vi "AUTON_Index.vi"(0 "Auton Array":dbl[][](array[numeric]), 5 "MeasuredHeading":dbl, 7 "LeftEncoder":dbl, 9 "RightEncoder":dbl, 11 "Kinect Array":dbl[](array[numeric])) -> (3 "Kinect Array Out":dbl[](array[numeric]), 4 "Left Drive":dbl, 6 "Right Drive":dbl)   [LabVIEW 2012]
uses:
  <vilib>/addons/Kinect/Skeleton Vertex Index.ctl
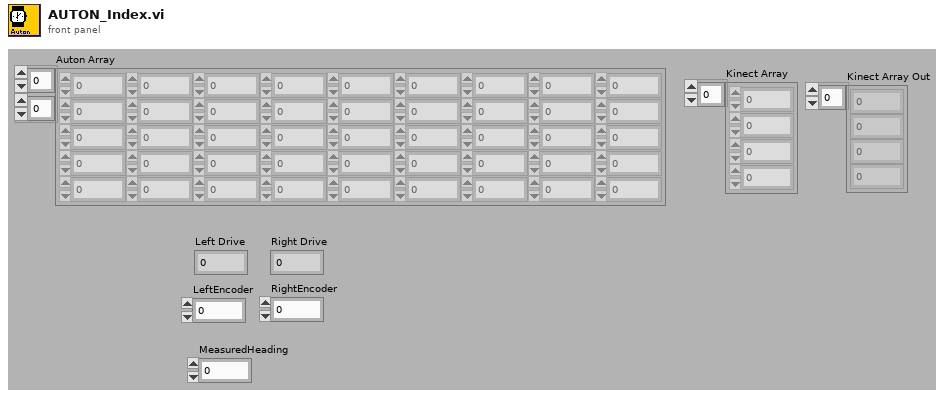
[diagram p1: front panel]
types:
  T1 = typedef "Skeleton Vertex Index.ctl" = i32
  T2 = cluster{"RightAxis":dbl, "LeftAxis":dbl, "RightHead":bool, "Left Head":bool, "Left Leg Out":bool, "Left Leg Forward":bool, "Left Leg Back":bool, "Right Leg Out":bool, "Right Leg Forward":bool, "Right Leg Back":bool}
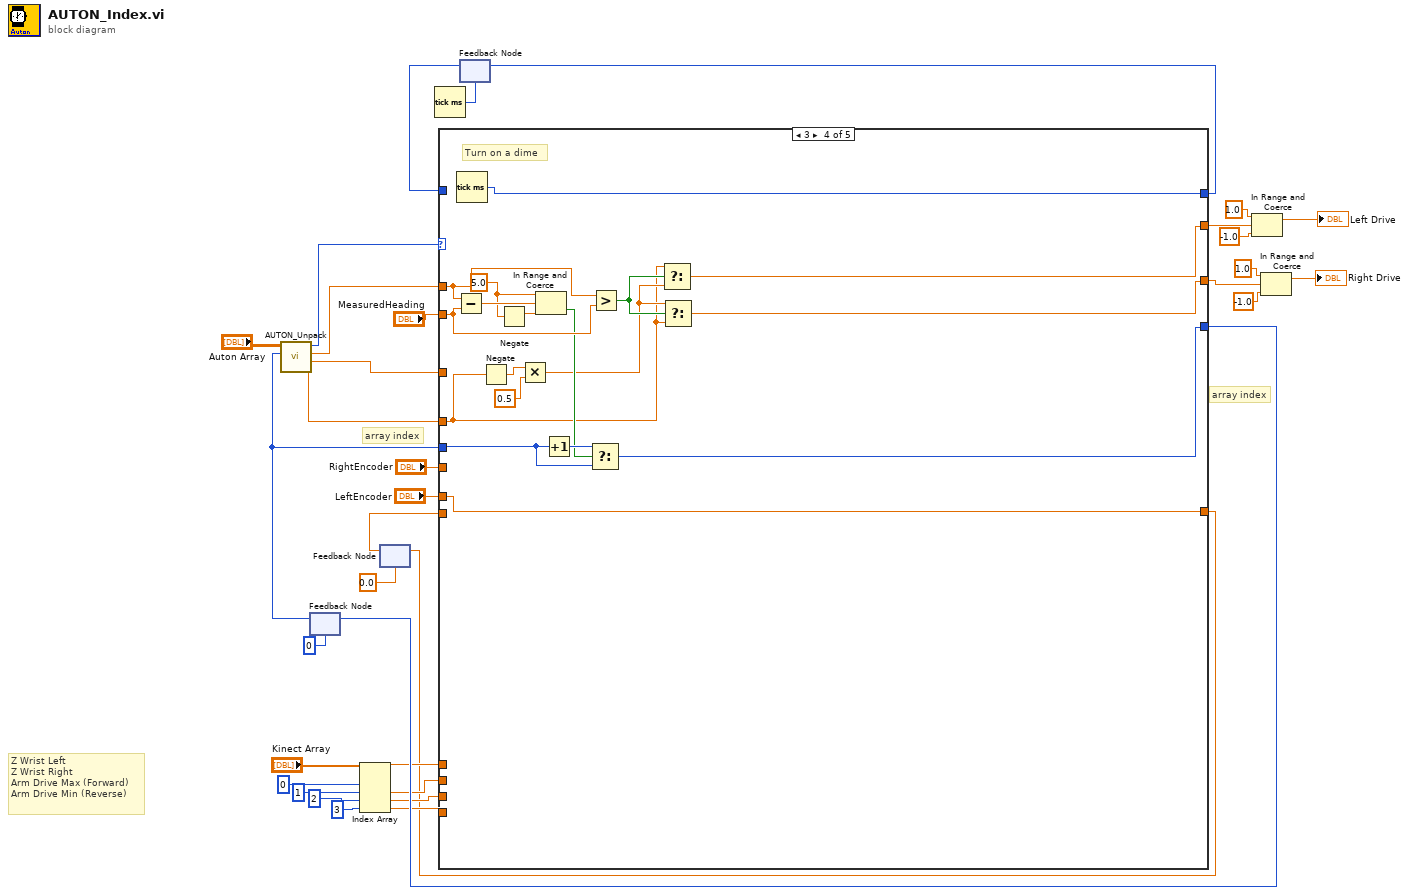
[diagram p0: block diagram]
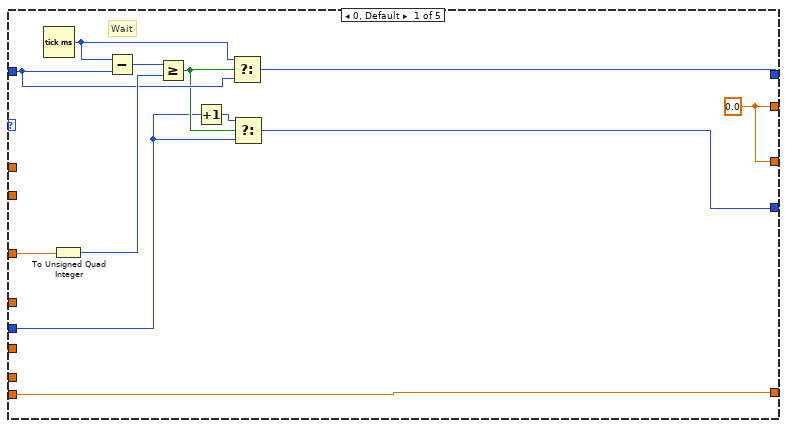
[diagram p2: hidden frame]
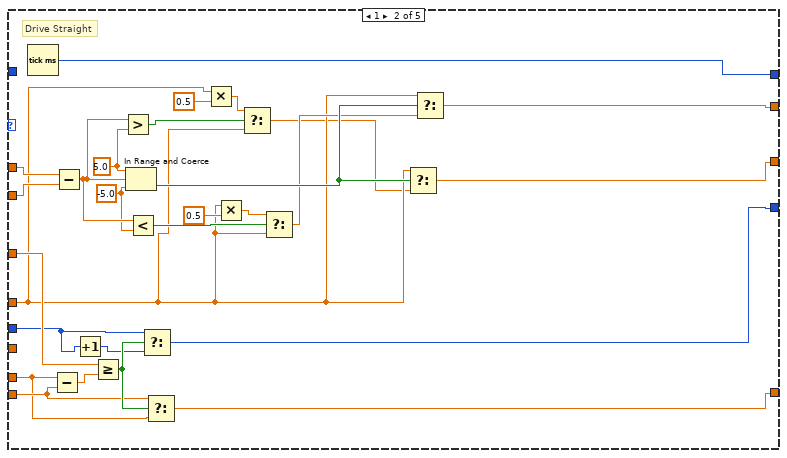
[diagram p3: hidden frame]
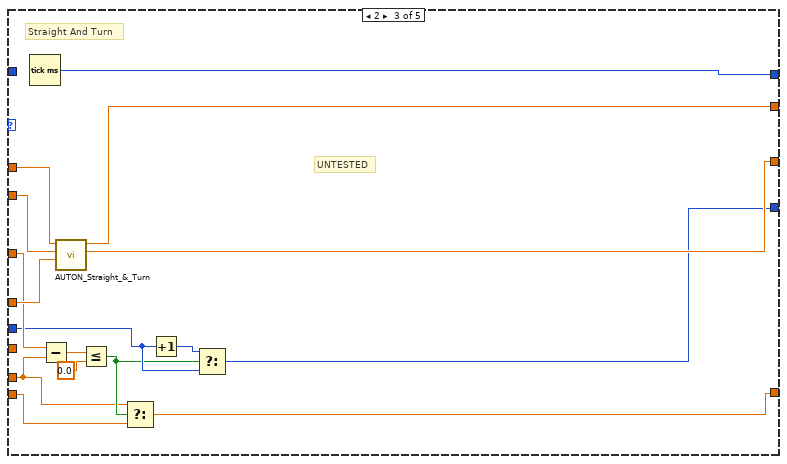
[diagram p4: hidden frame]
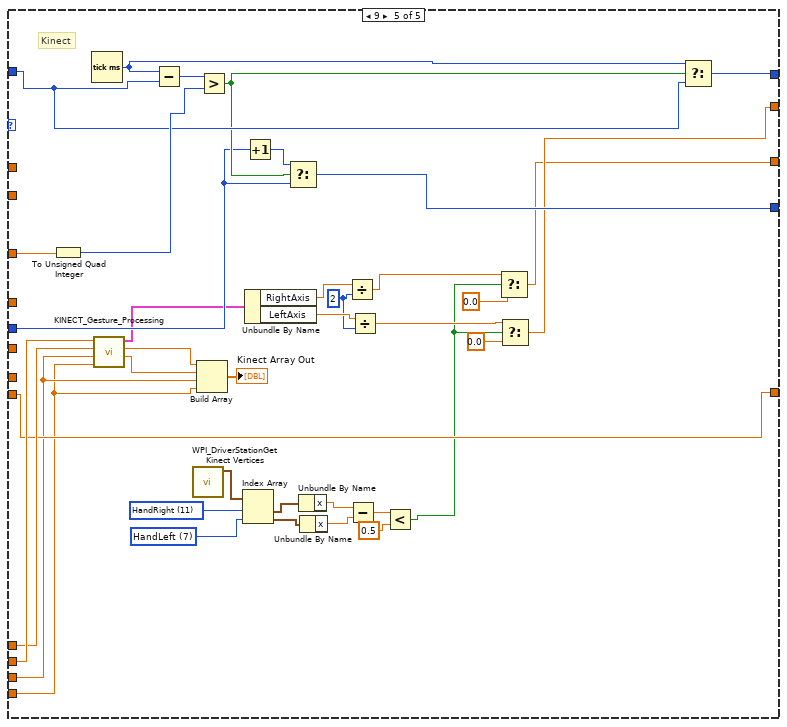
[diagram p5: hidden frame]
diagram:
  # "Z Wrist Left\nZ Wrist Right\nArm Drive Max (Forward)\nArm Drive Min (Reverse)"
  # "array index"
  # "array index"
  n1 = feedback #1(0) -> (w1:i32)
  n2 = call "AUTON_Unpack.vi"("Index"=w1, "all rows"="Auton Array") -> ("Power"=w4:dbl, "Time/Distance"=w2:dbl, "Desired Heading"=w3:dbl, "Primitive ID"=w5:i16)  [unwired: 4 in, 2 out]
  n3 = Index Array(array="Kinect Array", index #1=0 ("index"), index #2=1 ("index"), index #3=2 ("index"), index #4=3 ("index")) -> (element #1=w12:dbl, element #2=w11:dbl, element #3=w10:dbl, element #4=w9:dbl)
  n4 = feedback #2(0.0) -> (w7:dbl)
  n5 = Tick Count (ms)() -> (millisecond timer value=w31:u32)
  n6 = feedback #3(w31) -> (w33:u32)
  n7 = case shown="3" w5 {
    tunnel: [w38 w69 w78 w102 w137] -> w19
    tunnel: w1 -> [w39 w50 w79 w105 w138]
    tunnel: [w46 w47 w84 w107 w145] -> w21
    tunnel: w33 -> [w43 _ _ _ w142]
    tunnel: w2 -> [w36 w71 w83 _ w136]
    tunnel: w3 -> [_ w68 w89 w97 _]
    tunnel: [w37 w65 w86 w103 w127] -> w29
    tunnel: [w37 w64 w85 w104 w126] -> w22
    tunnel: w4 -> [_ w53 w87 w90 _]
    tunnel: "LeftEncoder" -> [_ w48 w75 w101 _]
    tunnel: "MeasuredHeading" -> [_ w67 w88 w96 _]
    tunnel: "RightEncoder" -> [_ _ _ _ _]
    tunnel: w12 -> [_ _ _ _ w115]
    tunnel: w11 -> [_ _ _ _ w116]
    tunnel: w10 -> [_ _ _ _ w111]
    tunnel: w9 -> [_ _ _ _ w110]
    tunnel: w7 -> [w35 w49 w76 _ w114]
    tunnel: [w35 w73 w74 w101 w114] -> w6
    frame 0, Default {
      w37 = 0.0 ("Numeric")
      # "Wait"
      n8 = Tick Count (ms)() -> (millisecond timer value=w42:u32)
      n9 = To Unsigned Quad Integer(1:w36) -> (0:w44:u64)
      n10 = Subtract(x=w42, y=w43) -> (x-y=w45:u32)
      n11 = Greater Or Equal?(x=w45, y=w44) -> (x >= y?=w41:bool)
      n12 = Increment(x=w39) -> (x+1=w40:i32)
      n13 = Select(t=w42, s=w41, f=w43) -> (s? t:f=w46:u32)
      n14 = Select(t=w40, s=w41, f=w39) -> (s? t:f=w38:i32)
    }
    frame 1 {
      w61 = -5.0 ("lower limit")
      w63 = 5.0 ("upper limit")
      # "Drive Straight"
      n15 = Tick Count (ms)() -> (millisecond timer value=w47:u32)
      n16 = Subtract(x=w48, y=w49) -> (x-y=w72:dbl)
      n17 = Subtract(x=w68, y=w67) -> (x-y=w62:dbl)
      n18 = Increment(x=w50) -> (x+1=w51:i32)
      n19 = Greater Or Equal?(x=w71, y=w72) -> (x >= y?=w70:bool)
      n20 = Greater?(x=w62, y=w63) -> (0:w56:bool)
      n21 = In Range and Coerce(upper limit=w63, x=w62, lower limit=w61) -> (In Range?=w66:bool)  [unwired: 1 out]
      n22 = Less?(x=w62, y=w61) -> (x < y?=w60:bool)
      n23 = Select(t=w50, s=w70, f=w51) -> (s? t:f=w69:i32)
      n24 = Select(t=w49, s=w70, f=w48) -> (s? t:f=w73:dbl)
      n25 = Multiply(x=w53, y=0.5) -> (x*y=w55:dbl)
      n26 = Multiply(x=w53, y=0.5) -> (x*y=w58:dbl)
      n27 = Select(t=w55, s=w56, f=w53) -> (s? t:f=w52:dbl)
      n28 = Select(t=w58, s=w60, f=w53) -> (s? t:f=w57:dbl)
      n29 = Select(t=w53, s=w66, f=w52) -> (s? t:f=w64:dbl)
      n30 = Select(t=w53, s=w66, f=w57) -> (s? t:f=w65:dbl)
    }
    frame 2 {
      # "UNTESTED"
      # "Straight And Turn"
      n31 = Tick Count (ms)() -> (millisecond timer value=w84:u32)
      n32 = Subtract(x=w83, y=w75) -> (x-y=w82:dbl)
      n33 = call "AUTON_Straight_&_Turn.vi"("Power"=w87, "Current Heading"=w88, "Desired Heading"=w89) -> ("Right Drive"=w85:dbl, "Left Drive"=w86:dbl)  [unwired: 7 in]
      n34 = Less Or Equal?(x=w82, y=0.0) -> (x <= y?=w77:bool)
      n35 = Select(t=w75, s=w77, f=w76) -> (s? t:f=w74:dbl)
      n36 = Increment(x=w79) -> (x+1=w80:i32)
      n37 = Select(t=w80, s=w77, f=w79) -> (s? t:f=w78:i32)
    }
    frame 3 {
      w98 = 5.0 ("upper limit")
      # "Turn on a dime"
      n38 = Subtract(x=w97, y=w96) -> (x-y=w100:dbl)
      n39 = Tick Count (ms)() -> (millisecond timer value=w107:u32)
      n40 = Negate(x=w90) -> (-x=w93:dbl)
      n41 = Negate(x=w98) -> (-x=w99:dbl)
      n42 = Multiply(x=w93, y=0.5) -> (x*y=w91:dbl)
      n43 = In Range and Coerce(upper limit=w98, x=w100, lower limit=w99) -> (In Range?=w95:bool)  [unwired: 1 out]
      n44 = Increment(x=w105) -> (x+1=w106:i32)
      n45 = Select(t=w106, s=w95, f=w105) -> (s? t:f=w102:i32)
      n46 = Greater?(x=w97, y=w96) -> (0:w94:bool)
      n47 = Select(t=w90, s=w94, f=w91) -> (s? t:f=w103:dbl)
      n48 = Select(t=w91, s=w94, f=w90) -> (s? t:f=w104:dbl)
    }
    frame 9 {
      w117 = T1 7 items=["HipCenter", "Spine", "ShoulderCenter", "Head", "ShoulderLeft", "ElbowLeft", "WristLeft", "HandLeft", "ShoulderRight", "ElbowRight", "WristRight", "HandRight", "HipLeft", "KneeLeft", "AnkleLeft", "FootLeft", "HipRight", "KneeRight", "AnkleRight", "FootRight"] ("Skeleton Joints")
      w119 = T1 11 items=["HipCenter", "Spine", "ShoulderCenter", "Head", "ShoulderLeft", "ElbowLeft", "WristLeft", "HandLeft", "ShoulderRight", "ElbowRight", "WristRight", "HandRight", "HipLeft", "KneeLeft", "AnkleLeft", "FootLeft", "HipRight", "KneeRight", "AnkleRight", "FootRight"] ("Skeleton Joints")
      w132 = 2
      # "Kinect"
      n49 = To Unsigned Quad Integer(1:w136) -> (0:w143:u64)
      n50 = Tick Count (ms)() -> (millisecond timer value=w141:u32)
      n51 = call "KINECT_Gesture_Processing.vi"("Z Wrist Right in"=w116, "Z Wrist Left in"=w115, "Arm Drive in Max (Forward)"=w111, "Arm Drive in Min (Reverse)"=w110) -> ("Joystick Data"=w135:T2, "Z Wrist Right out"=w113:dbl, "Z Wrist Left out"=w112:dbl)  [unwired: 2 in]
      n52 = Subtract(x=w141, y=w142) -> (x-y=w144:u32)
      n53 = call <vilib>:"WPI_DriverStationGet Kinect Vertices.vi"() -> ("Skeleton Vertices"=w125:cluster{"x":sgl, "y":sgl, "z":sgl}[])  [unwired: 10 in, 1 out]
      n54 = Build Array(w113, w112, w111, w110) -> (→"Kinect Array Out":dbl[])
      n55 = Greater?(x=w144, y=w143) -> (0:w140:bool)
      n56 = Index Array(array=w125, index #1=w119, index #2=w117) -> (element #1=w120:cluster{"x":sgl, "y":sgl, "z":sgl}, element #2=w118:cluster{"x":sgl, "y":sgl, "z":sgl})
      n57 = Increment(x=w138) -> (x+1=w139:i32)
      n58 = Unbundle By Name(w135) -> ("RightAxis"=w134:dbl, "LeftAxis"=w133:dbl)
      n59 = Select(t=w139, s=w140, f=w138) -> (s? t:f=w137:i32)
      n60 = Unbundle By Name(w120) -> ("x"=w124:sgl)
      n61 = Unbundle By Name(w118) -> ("x"=w123:sgl)
      n62 = Divide(x=w134, y=w132) -> (x/y=w131:dbl)
      n63 = Subtract(x=w124, y=w123) -> (x-y=w122:sgl)
      n64 = Divide(x=w133, y=w132) -> (x/y=w130:dbl)
      n65 = Less?(x=w122, y=sgl 0.5) -> (x < y?=w108:bool)
      n66 = Select(t=w131, s=w108, f=0.0) -> (s? t:f=w126:dbl)
      n67 = Select(t=w130, s=w108, f=0.0) -> (s? t:f=w127:dbl)
      n68 = Select(t=w141, s=w140, f=w142) -> (s? t:f=w145:u32)
    }
  }
  n69 = feedback-in #1(w19) -> ()
  n70 = feedback-in #2(w6) -> ()
  n71 = feedback-in #3(w21) -> ()
  n72 = In Range and Coerce(upper limit=1.0, x=w29, lower limit=-1.0) -> (coerced(x)=→"Left Drive":dbl)  [unwired: 1 out]
  n73 = In Range and Coerce(upper limit=1.0, x=w22, lower limit=-1.0) -> (coerced(x)=→"Right Drive":dbl)  [unwired: 1 out]
